vi "Open and Add Reply Protocol.vi"(8 "Error In":errorcluster, 10 "Reply Protocol Base":refnum<class "Reply Protocol Base.lvclass">, 11 "reference in":refnum<class "Reply Protocol Manager.lvclass">) -> (0 "Error Out":errorcluster, 3 "reference out":refnum<class "Reply Protocol Manager.lvclass">)   [LabVIEW 2023, in "HAL GOOP4.lvlib" / "Reply Protocol Manager.lvclass"]
uses:
  Reply Protocol Manager.lvclass
  Reply Protocol/Reply Protocol Base/Reply Protocol Base.lvclass
  Reply Protocol/Reply Protocol Base/Reply Protocol Base.lvclass/Reply Protocol Base.ctl
  Reply Protocol Manager.lvclass/Reply Protocol Manager.ctl
  <vilib>/Utility/miscctls.llb/LVMapReplaceAction.ctl
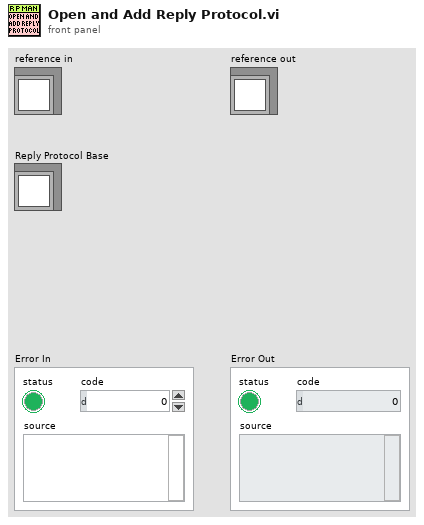
[diagram p1: front panel]
types:
  T1 = typedef "LVMapReplaceAction.ctl" = enum32{"Modify Entry only if found", "Add or Modify Entry", "Delete Entry"}
  T2 = typedef "HAL GOOP4.lvlib/Reply Protocol Manager.lvclass/ObjectAttributes.ctl" = cluster{"Reply Protocols":map{string, refnum<class "Reply Protocol Base.lvclass">}}
  T3 = map{string, refnum<class "Reply Protocol Base.lvclass">}
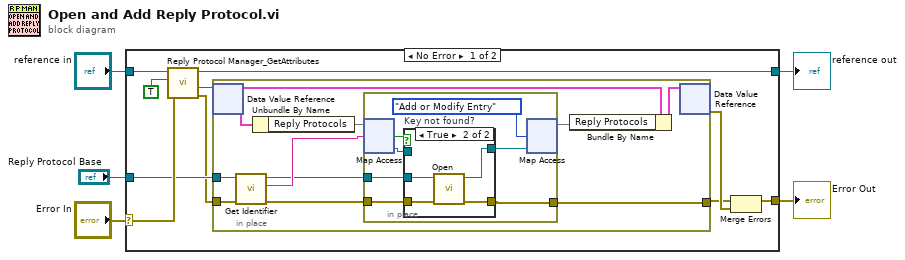
[diagram p0: block diagram]
diagram:
  n1 = case shown="No Error" "Error In" {
    selector: "Error In" -> [w14 w39]
    tunnel: [w11 w39] -> w4
    tunnel: [w12 w38] -> w2
    tunnel: "reference in" -> [w15 w38]
    tunnel: "Reply Protocol Base" -> [w8 _]
    frame No Error {
      n2 = call "Reply Protocol Manager_GetAttributes.vi"("Error In"=w14, "OnlyGetDvrReference(False)"=TRUE, "reference in"=w15) -> ("Error Out"=w7:errorcluster, "DataRef"=w10:refnum<data-value>, "reference out"=w12:refnum<class "Reply Protocol Manager.lvclass">)  [unwired: 5 in, 1 out]
      n3 = in-place {
        in-place-border: w8 -> [w22]
        in-place-border: w7 -> [w19]
        in-place-border: [w17] -> w6
        n4 = in-place-dvr #1(w10) -> (w23:T2)  [unwired: 1 out]
        n5 = call "Get Identifier.vi"("Reply Protocol Base in"=w22) -> ("Identifier"=w20:string, "Reply Protocol Base out"=w18:refnum<class "Reply Protocol Base.lvclass">)  [unwired: 9 in]
        n6 = Unbundle By Name(w23) -> ("Reply Protocols"=w21:T3)
        n7 = in-place {
          in-place-border: w19 -> [w30]
          in-place-border: w18 -> [w29]
          in-place-border: [w25] -> w17
          n8 = in-place-map #2(w21, w20) -> (w26:refnum<class "Reply Protocol Base.lvclass">, w31:bool)  [unwired: 1 in]
          n9 = case "Key not found?" shown="True" w31 {
            tunnel: w30 -> [w33 w37]
            tunnel: w29 -> [_ w36]
            tunnel: [w33 w35] -> w25
            tunnel: [w32 w34] -> w27
            tunnel: w26 -> [w32 _]
            frame False {
            }
            frame True {
              n10 = call-dynamic "Open.vi"("error in"=w37, "Reply Protocol in"=w36) -> ("error out"=w35:errorcluster, "Reply Protocol out"=w34:refnum<class "Reply Protocol Base.lvclass">)  [unwired: 8 in]
            }
          }
          n11 = in-place-map #2(w27, LVMapReplaceAction."Add or Modify Entry" ("action")) -> (w16:T3)  [unwired: 2 out]
        }
        n12 = Bundle By Name(cluster=w23, "Reply Protocols"=w16) -> (w24:T2)
        n13 = in-place-dvr #1(w24) -> (w13:errorcluster)  [unwired: 1 out]
      }
      n14 = Merge Errors(w6, w13) -> (w11:errorcluster)
    }
    frame Error {
    }
  }
  "Error Out" <- w4
  "reference out" <- w2
